vi "Drive Logic.vi"(1 "Drive Info  In":T1) -> (0 "Drive Info Out":T1)   [LabVIEW 2013]
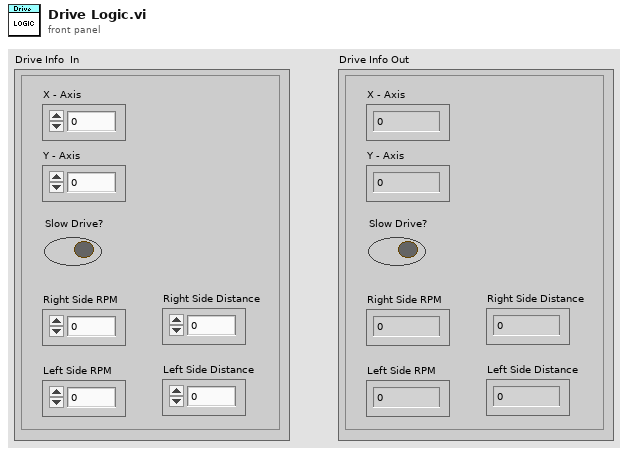
[diagram p1: front panel]
types:
  T1 = cluster{"X - Axis":dbl, "Y - Axis":dbl, "Slow Drive?":bool, "Right Side RPM":dbl, "Right Side Distance":dbl, "Left Side RPM ":dbl, "Left Side Distance":dbl}
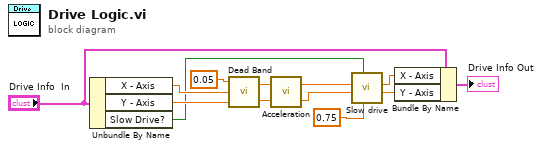
[diagram p0: block diagram]
diagram:
  n1 = Unbundle By Name("Drive Info  In") -> ("X - Axis"=w12:dbl, "Y - Axis"=w11:dbl, "Slow Drive?"=w8:bool)
  n2 = call "Dead Band.vi"("Axis 2 In"=w11, "Axis 1 In"=w12, "Dead Band"=0.05) -> ("Axis 2 Out"=w9:dbl, "Axis 1 Out"=w10:dbl)
  n3 = call "Acceleration.vi"("Y Input"=w9, "X Input"=w10) -> ("Y Output"=w6:dbl, "X Output"=w7:dbl)
  n4 = call "Slow drive.vi"("Slow drive to"=0.75, "Slow?"=w8, "Y-Axis"=w6, "X-Axis"=w7) -> ("Y - Axis out"=w1:dbl, "X-Axis out"=w2:dbl)  [unwired: 6 in]
  n5 = Bundle By Name(cluster="Drive Info  In", "X - Axis"=w2, "Y - Axis"=w1) -> (→"Drive Info Out":T1)
